vi "Close Project.vi"(8 "error in":errorcluster, 11 "Project ref":refnum<vi>) -> (0 "error out":errorcluster)   [LabVIEW 2020, in "MeasurementService Editor.lvlib"]
uses:
  MeasurementService Editor.lvlib
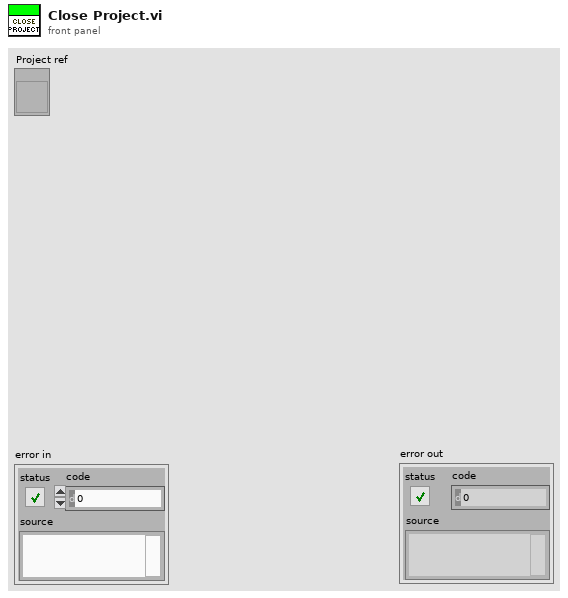
[diagram p1: front panel]
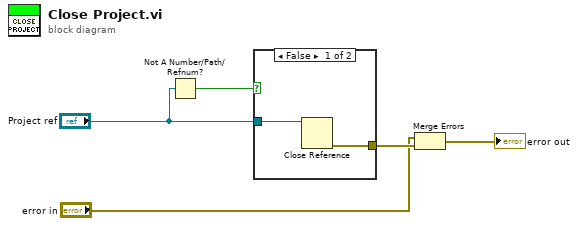
[diagram p0: block diagram]
diagram:
  n1 = Not A Number/Path/Refnum?(number/path/refnum="Project ref") -> (NaN/Path/Refnum?=w1:bool)
  n2 = case shown="False" w1 {
    tunnel: [w7 _] -> w5
    tunnel: "Project ref" -> [w6 _]
    frame False {
      n3 = Close Reference(reference=w6) -> (error out=w7:errorcluster)  [unwired: 1 in]
    }
    frame True {
    }
  }
  n4 = Merge Errors("error in", w5) -> (→"error out":errorcluster)
